vi "Generate Dummy Digitizer Corrections Files.vi"(8 "error in":errorcluster, 11 "TWM pipe":string="\\\\.\\pipe\\TWM:server") -> (0 "error out":errorcluster)   [LabVIEW 2020]
uses:
  <vilib>/Utility/error.llb/DialogType.ctl
  external libraries/TWM client.lvlibp
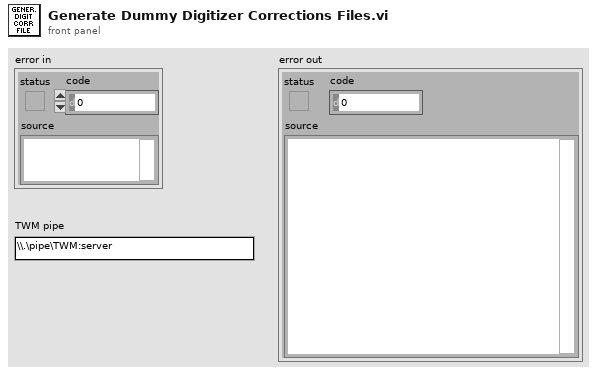
[diagram p1: front panel]
types:
  T1 = typedef "DialogType.ctl" = u16
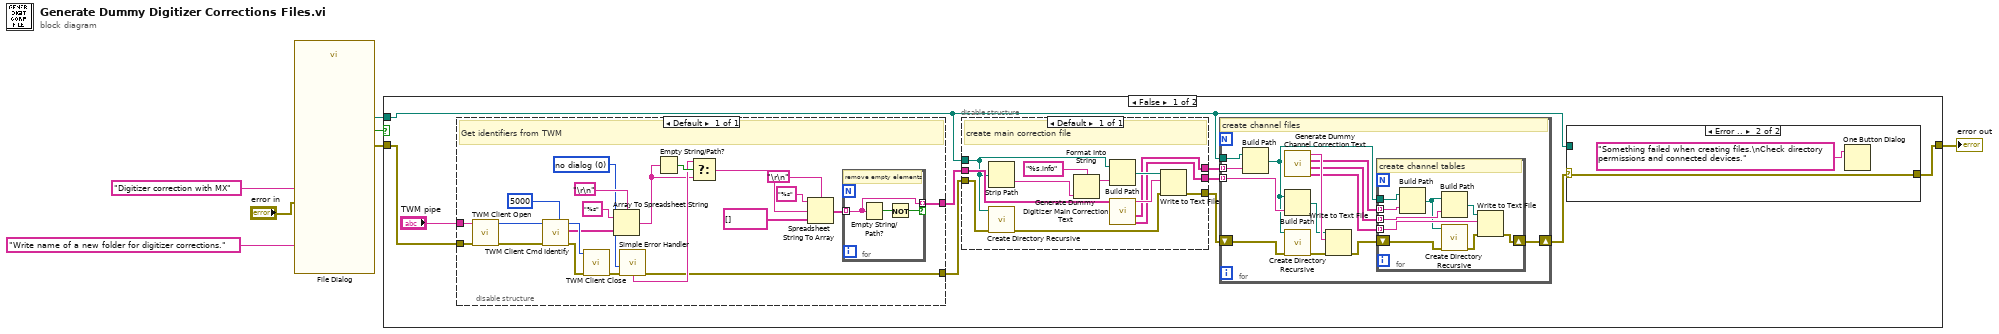
[diagram p0: block diagram]
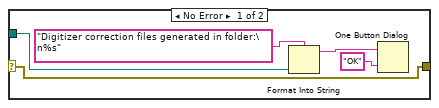
[diagram p2: hidden frame]
diagram:
  n1 = call "File Dialog"("prompt"="Write name of a new folder for digitizer corrections.", "default name"="Digitizer correction with MX", "error in"="error in") -> ("selected path"=w1:path, "cancelled"=w4:bool, "error out"=w3:errorcluster)  [unwired: 9 in, 1 out]
  n2 = case shown="False" w4 {
    tunnel: [w11 w84] -> w2
    tunnel: w3 -> [w9 w84]
    tunnel: w1 -> [w10 _]
    frame False {
      n3 = disable-structure shown="Default" {
        disable-tunnel: "TWM pipe" -> [w68]
        disable-tunnel: [w61] -> w17
        disable-tunnel: w9 -> [w60]
        disable-tunnel: [w59] -> w8
        frame Enabled {
          w72 = T1 0 items=["no dialog", "OK message", "continue or stop message", "OK message + warnings", "continue/stop + warnings"] ("type of dialog (OK msg:1)")
          # "Get identifiers from TWM"
          n4 = call "TWM Client Open.vi"("error in"=w60, "pipe name"=w68) -> ("error out"=w79:errorcluster, "handle out"=w78:i32)  [unwired: 8 in]
          n5 = call "TWM Client Cmd Identify.vi"("timeout [ms]"=5000, "error in"=w79, "handle"=w78) -> ("error out"=w80:errorcluster, "channel idns"=w67:string[], "handle out"=w77:i32)  [unwired: 5 in, 1 out]
          n6 = call "TWM Client Close.vi"("error in"=w80, "handle in"=w77) -> ("error out"=w73:errorcluster)  [unwired: 9 in]
          n7 = Array To Spreadsheet String(delimiter (Tab)="\r\n", array=w67, 3:"%s" ("format string")) -> (spreadsheet string=w69:string)
          n8 = call <vilib>:"Simple Error Handler.vi"("type of dialog (OK msg:1)"=w72, "error in (no error)"=w73) -> ("error out"=w59:errorcluster, "message"=w70:string)  [unwired: 3 in, 3 out]
          n9 = Empty String/Path?(string/path=w69) -> (empty?=w71:bool)
          n10 = Select(t=w70, s=w71, f=w69) -> (s? t:f=w66:string)
          n11 = Spreadsheet String To Array(delimiter (Tab)="\r\n", format string="%s", spreadsheet string=w66, array type (2D Dbl)=string[] [] ("appended array")) -> (array=w62:string[])
          n12 = for {
            tunnel: w62 -> [w83] mode=indexing
            tunnel: [w83] -> w61 mode=indexing if=w81
            # "remove empty elements"
            n13 = Empty String/Path?(string/path=w83) -> (empty?=w82:bool)
            n14 = Not(x=w82) -> (.not. x?=w81:bool)
          }
        }
      }
      n15 = disable-structure shown="Default" {
        disable-tunnel: w17 -> [w36]
        disable-tunnel: [w30] -> w15
        disable-tunnel: [w29] -> w14
        disable-tunnel: w10 -> [w27]
        disable-tunnel: w8 -> [w26]
        disable-tunnel: [w28] -> w13
        frame Enabled {
          # "create main correction file"
          n16 = Strip Path(path=w27) -> (name=w34:string)  [unwired: 1 out]
          n17 = call <vilib>:"Create Directory Recursive.vi"("error in (no error)"=w26, "directory"=w27) -> ("error out"=w25:errorcluster)  [unwired: 3 in, 2 out]
          n18 = Format Into String(format string="%s.info", w34) -> (resulting string=w32:string)  [unwired: 2 in, 1 out]
          n19 = Build Path(base path=w27, name or relative path=w32) -> (appended path=w31:path)
          n20 = call "Generate Dummy Digitizer Main Correction Text.vi"("Digitizer identifications"=w36) -> ("Channels file names"=w28:string[], "Channels directories"=w29:string[], "main digitizer correction info file"=w35:string)  [unwired: 8 in]
          n21 = Write to Text File(file (use dialog)=w31, text=w35, error in=w25) -> (error out=w30:errorcluster)  [unwired: 1 in, 2 out]
        }
      }
      n22 = for {
        shift-right: [w41] -> w12
        shift-left: w15 -> [w38]
        tunnel: w10 -> [w49]
        tunnel: w14 -> [w48] mode=indexing
        tunnel: w13 -> [w47] mode=indexing
        # "create channel files"
        n23 = Build Path(base path=w49, name or relative path=w48) -> (appended path=w39:path)
        n24 = call "Generate Dummy Channel Correction Text.vi"() -> ("Tables"=w43:string[], "Tables filenames"=w44:string[], "Tables directories"=w45:string[], "Channel correction file"=w46:string)  [unwired: 8 in]
        n25 = Build Path(base path=w39, name or relative path=w47) -> (appended path=w40:path)
        n26 = call <vilib>:"Create Directory Recursive.vi"("error in (no error)"=w38, "directory"=w39) -> ("error out"=w37:errorcluster)  [unwired: 3 in, 2 out]
        n27 = Write to Text File(file (use dialog)=w40, text=w46, error in=w37) -> (error out=w42:errorcluster)  [unwired: 1 in, 2 out]
        n28 = for {
          tunnel: w39 -> [w58]
          tunnel: w45 -> [w57] mode=indexing
          tunnel: w44 -> [w56] mode=indexing
          tunnel: w43 -> [w54] mode=indexing
          shift-right: [w53] -> w41
          shift-left: w42 -> [w51]
          # "create channel tables"
          n29 = Build Path(base path=w58, name or relative path=w57) -> (appended path=w50:path)
          n30 = Build Path(base path=w50, name or relative path=w56) -> (appended path=w55:path)
          n31 = call <vilib>:"Create Directory Recursive.vi"("error in (no error)"=w51, "directory"=w50) -> ("error out"=w52:errorcluster)  [unwired: 3 in, 2 out]
          n32 = Write to Text File(file (use dialog)=w55, text=w54, error in=w52) -> (error out=w53:errorcluster)  [unwired: 1 in, 2 out]
        }
      }
      n33 = case shown="Error .." w12 {
        selector: w12 -> [w22 w23]
        tunnel: [w22 w23] -> w11
        tunnel: w10 -> [w20 _]
        frame No Error {
          n34 = Format Into String(format string="Digitizer correction files generated in folder:\n%s", w20) -> (resulting string=w19:string)  [unwired: 2 in, 1 out]
          n35 = One Button Dialog(message=w19, button name ("OK")="OK") -> ()  [unwired: 1 out]
        }
        frame Error {
          n36 = One Button Dialog(message="Something failed when creating files.\nCheck directory permissions and connected devices.") -> ()  [unwired: 1 in, 1 out]
        }
      }
    }
    frame True {
    }
  }
  "error out" <- w2
